vi "Array Enum Page.vi"() -> ()   [LabVIEW 2019]
panel:
  out "Element Page 2":T1
  out "Element Page 1":T1
  out "Element Main":T1
  out "Enum Main":T2(ring)
  in  "Output":T3(array[cluster])
  in  "Tab Control":enum32{"Main", "Page 1", "Page 2"}(tab)
  in  "Main":T3(array[cluster])
  in  "Page 1":T3(array[cluster])
  in  "Page 2":T3(array[cluster])
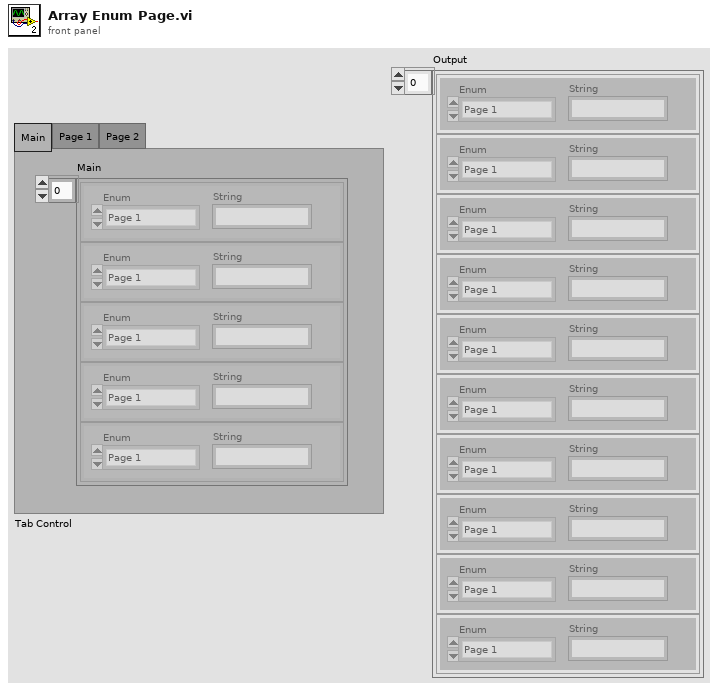
[diagram p1: front panel]
types:
  T1 = cluster{"Enum":enum16{"Page 1", "Page 2", "Qrcode Main", "Qrcode Page 1", "Qrcode Page 2"}, "String":string}
  T2 = enum16{"Page 1", "Page 2", "Qrcode Main", "Qrcode Page 1", "Qrcode Page 2"}
  T3 = cluster{"Enum":enum16{"Page 1", "Page 2", "Qrcode Main", "Qrcode Page 1", "Qrcode Page 2"}, "String":string}[]
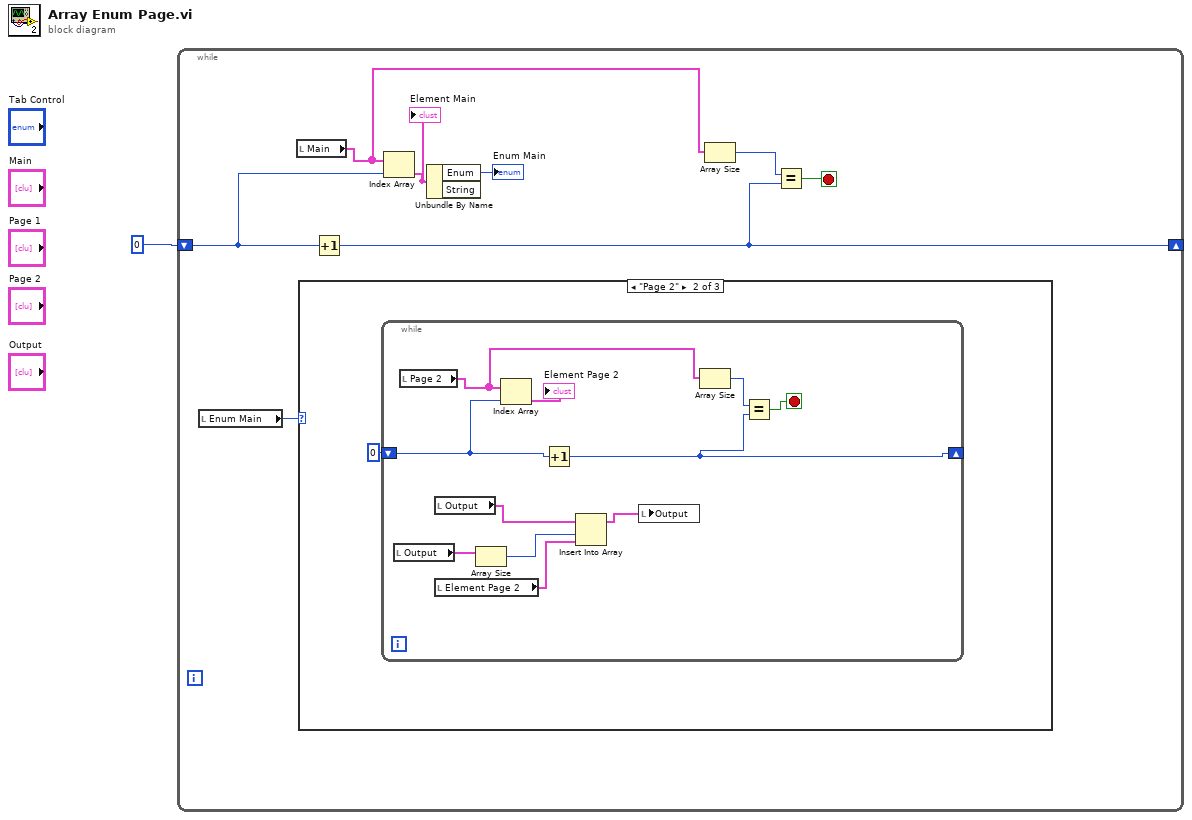
[diagram p0: block diagram]
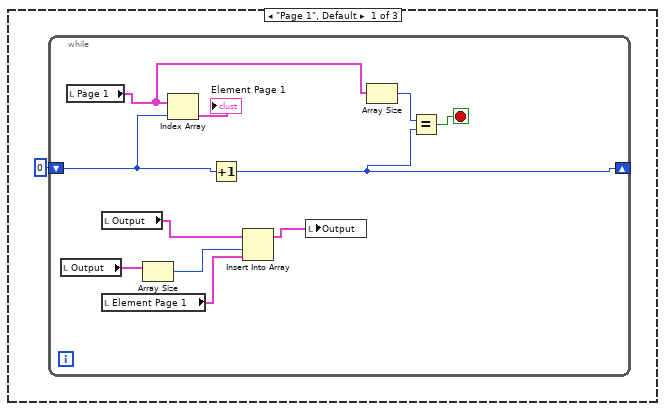
[diagram p2: hidden frame]
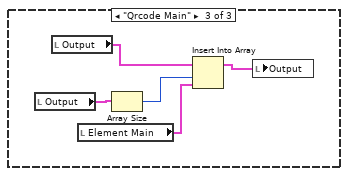
[diagram p3: hidden frame]
diagram:
  n1 = while {
    shift-right: [w4] -> _
    shift-left: 0 -> [w9]
    stop <- w3 stop-if-true
    n2 = local read "Enum Main"() -> (w2:T2)
    n3 = local read "Main"() -> (w6:T3)
    n4 = case shown="\"Page 2\"" w2 {
      frame "Page 1", Default {
        n5 = while {
          shift-right: [w13] -> _
          shift-left: 0 -> [w20]
          stop <- w11 stop-if-true
          n6 = local read "Output"() -> (w18:T3)
          n7 = local read "Page 1"() -> (w14:T3)
          n8 = local read "Output"() -> (w21:T3)
          n9 = local read "Element Page 1"() -> (w16:T1)
          n10 = Array Size(array=w18) -> (size(s)=w17:i32)
          n11 = Index Array(array=w14, index=w20) -> (element=→"Element Page 1":T1)
          n12 = Increment(x=w20) -> (x+1=w13:i32)
          n13 = Insert Into Array(array=w21, index=w17, new element=w16) -> (w15:T3)
          n14 = local write "Output"(w15) -> ()
          n15 = Array Size(array=w14) -> (size(s)=w12:i32)
          n16 = Equal?(x=w12, y=w13) -> (x = y?=w11:bool)
        }
      }
      frame "Page 2" {
        n17 = while {
          shift-right: [w25] -> _
          shift-left: 0 -> [w32]
          stop <- w23 stop-if-true
          n18 = local read "Output"() -> (w30:T3)
          n19 = local read "Page 2"() -> (w26:T3)
          n20 = local read "Output"() -> (w33:T3)
          n21 = local read "Element Page 2"() -> (w28:T1)
          n22 = Array Size(array=w30) -> (size(s)=w29:i32)
          n23 = Index Array(array=w26, index=w32) -> (element=→"Element Page 2":T1)
          n24 = Increment(x=w32) -> (x+1=w25:i32)
          n25 = Insert Into Array(array=w33, index=w29, new element=w28) -> (w27:T3)
          n26 = local write "Output"(w27) -> ()
          n27 = Array Size(array=w26) -> (size(s)=w24:i32)
          n28 = Equal?(x=w24, y=w25) -> (x = y?=w23:bool)
        }
      }
      frame "Qrcode Main" {
        n29 = local read "Output"() -> (w37:T3)
        n30 = local read "Output"() -> (w38:T3)
        n31 = local read "Element Main"() -> (w35:T1)
        n32 = Array Size(array=w37) -> (size(s)=w36:i32)
        n33 = Insert Into Array(array=w38, index=w36, new element=w35) -> (w34:T3)
        n34 = local write "Output"(w34) -> ()
      }
    }
    n35 = Increment(x=w9) -> (x+1=w4:i32)
    n36 = Index Array(array=w6, index=w9) -> (element=w8:T1)
    "Element Main" <- w8
    n37 = Unbundle By Name(w8) -> ("Enum"=→"Enum Main":T2)  [unwired: 1 out]
    n38 = Array Size(array=w6) -> (size(s)=w5:i32)
    n39 = Equal?(x=w5, y=w4) -> (x = y?=w3:bool)
  }
